vi "Recieve Response with Result.vi"(4 "Finished":bool=TRUE, 6 "Result":refnum<class "Mag Lab Result.lvclass">, 8 "error in (no error)":errorcluster, 9 "Requestor":string, 10 "Requestee":string, 11 "Sequence Stepper in":refnum<class "Sequence Stepper.lvclass">) -> (0 "error out":errorcluster, 3 "Sequence Stepper out":refnum<class "Sequence Stepper.lvclass">)   [LabVIEW 2015, in "Sequence Stepper.lvclass"]
uses:
  Sequence Stepper.lvclass
  Mag Lab Result/Mag Lab Result.lvclass
  Mag Lab Root/Mag Lab Root.lvclass/Mag Lab Root.ctl
  <vilib>/ActorFramework/Actor/Actor.lvclass/Actor.ctl
  Sequence Stepper.lvclass/Sequence Stepper.ctl
  Stepper stage.ctl
  Mag Lab Root Messages/Set Output Msg/Recieve Set Output Msg.lvclass/Recieve Set Output Msg.ctl
  <vilib>/ActorFramework/Message Enqueuer/Message Enqueuer.lvclass/Message Enqueuer.ctl
  <vilib>/ActorFramework/Message Enqueuer/Enqueue.vi
  <vilib>/ActorFramework/Message Priority Queue/Priority Enqueue.vi
  Mag Lab Root Messages/Set Output Msg/Recieve Set Output Msg.lvclass
  Hardware/Source/Settle output/Settle Output.lvclass
  Stepping Function/Stepping Function.lvclass
  Mag Lab Root/Mag Lab Root.lvclass
  <vilib>/ActorFramework/Actor/Actor.lvclass
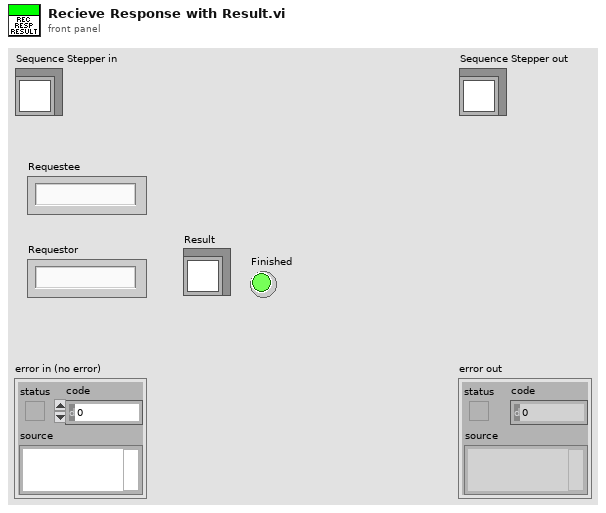
[diagram p1: front panel]
types:
  T1 = typedef "Stepper stage.ctl" = enum16{"New step", "Waiting to settle"}
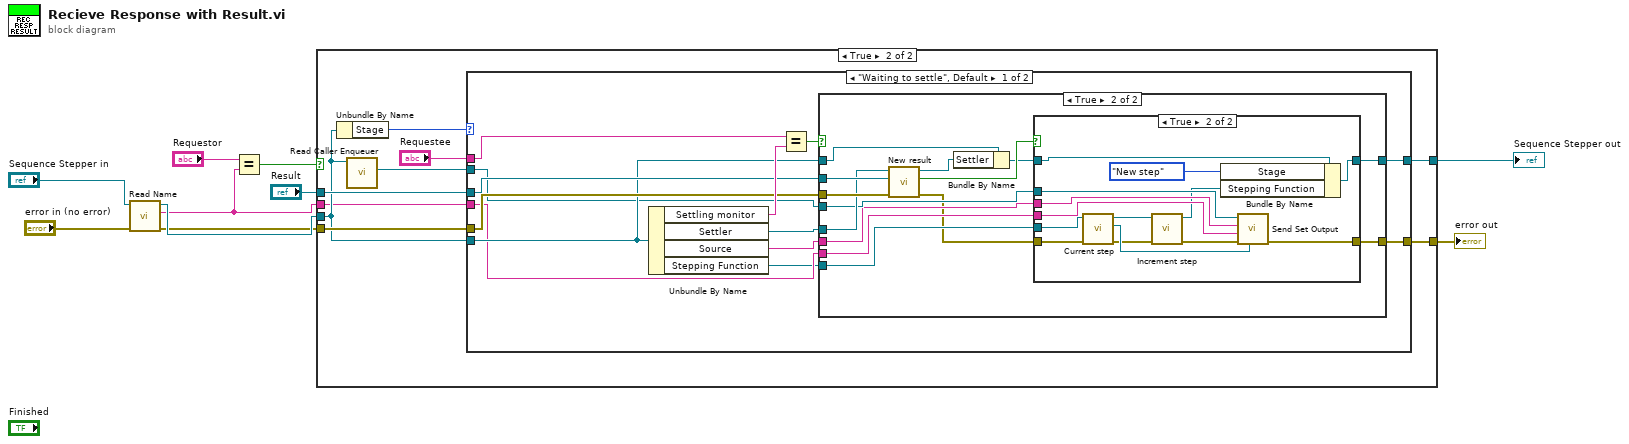
[diagram p0: block diagram]
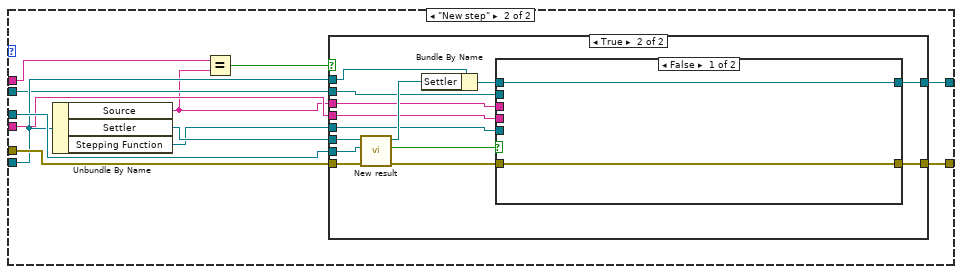
[diagram p5: hidden frame]
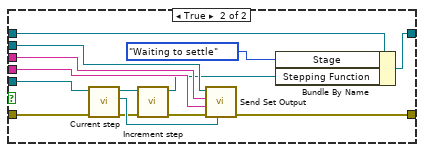
[diagram p7: hidden frame]
diagram:
  n1 = call "Read Name.vi"("error in (no error)"="error in (no error)", "Mag Lab Root in"="Sequence Stepper in") -> ("error out"=w5:errorcluster, "Name"=w3:string, "Mag Lab Root out"=w7:refnum<class "Sequence Stepper.lvclass">)  [unwired: 7 in]
  n2 = Equal?(x="Requestor", y=w3) -> (x = y?=w8:bool)
  n3 = case shown="True" w8 {
    tunnel: w7 -> [w12 w17]
    tunnel: "Result" -> [_ w19]
    tunnel: w5 -> [w11 w18]
    tunnel: w3 -> [_ w15]
    tunnel: [w12 w14] -> w2
    tunnel: [w11 w13] -> w1
    frame False {
    }
    frame True {
      n4 = Unbundle By Name(w17) -> ("Stage"=w21:T1)
      n5 = call <vilib>:"Read Caller Enqueuer.vi"("Actor"=w17) -> ("Caller Enqueuer"=w16:refnum<class "Message Enqueuer.lvclass">)  [unwired: 10 in]
      n6 = case shown="\"Waiting to settle\", Default" w21 {
        tunnel: "Requestee" -> [w34 w78]
        tunnel: w17 -> [w29 w74]
        tunnel: w19 -> [w32 w77]
        tunnel: w18 -> [w31 w76]
        tunnel: w16 -> [w27 w72]
        tunnel: w15 -> [w26 w71]
        tunnel: [w23 w69] -> w14
        tunnel: [w22 w68] -> w13
        frame "Waiting to settle", Default {
          n7 = Unbundle By Name(w29) -> ("Settling monitor"=w33:string, "Settler"=w28:refnum<class "Settle Output.lvclass">, "Source"=w25:string, "Stepping Function"=w24:refnum<class "Stepping Function.lvclass">)
          n8 = Equal?(x=w34, y=w33) -> (x = y?=w30:bool)
          n9 = case shown="True" w30 {
            tunnel: w32 -> [_ w50]
            tunnel: w31 -> [w35 w49]
            tunnel: w29 -> [w36 w48]
            tunnel: w28 -> [_ w46]
            tunnel: w27 -> [_ w43]
            tunnel: w26 -> [_ w42]
            tunnel: w25 -> [_ w41]
            tunnel: w24 -> [_ w40]
            tunnel: [w36 w38] -> w23
            tunnel: [w35 w37] -> w22
            frame False {
            }
            frame True {
              n10 = call-dynamic "New result.vi"("error in (no error)"=w49, "Result"=w50, "Settle Output in"=w46) -> ("error out"=w39:errorcluster, "Is output settled?"=w45:bool, "Settle Output out"=w47:refnum<class "Settle Output.lvclass">)  [unwired: 6 in]
              n11 = Bundle By Name(cluster=w48, "Settler"=w47) -> (w44:refnum<class "Sequence Stepper.lvclass">)
              n12 = case shown="True" w45 {
                tunnel: w44 -> [w52 w66]
                tunnel: w43 -> [_ w64]
                tunnel: w42 -> [_ w62]
                tunnel: w41 -> [_ w63]
                tunnel: w40 -> [_ w61]
                tunnel: w39 -> [w51 w55]
                tunnel: [w52 w54] -> w38
                tunnel: [w51 w53] -> w37
                frame False {
                }
                frame True {
                  n13 = call-dynamic "Current step.vi"("error in (no error)"=w55, "Stepping Function in"=w61) -> ("error out"=w57:errorcluster, "Step value"=w59:refnum<class "Mag Lab Result.lvclass">, "Stepping Function out"=w60:refnum<class "Stepping Function.lvclass">)  [unwired: 7 in]
                  n14 = call-dynamic "Increment step.vi"("error in (no error)"=w57, "Stepping Function in"=w60) -> ("error out"=w56:errorcluster, "Stepping Function out"=w58:refnum<class "Stepping Function.lvclass">)  [unwired: 8 in]
                  n15 = Bundle By Name(cluster=w66, "Stage"=Stepper_stage."New step", "Stepping Function"=w58) -> (w54:refnum<class "Sequence Stepper.lvclass">)
                  n16 = call "Send Set Output.vi"("Output value"=w59, "error in (no error)"=w56, "Requestor"=w62, "Requestee"=w63, "Message Enqueuer"=w64) -> ("error out"=w53:errorcluster)  [unwired: 5 in, 1 out]
                }
              }
            }
          }
        }
        frame "New step" {
          n17 = Unbundle By Name(w74) -> ("Source"=w67:string, "Settler"=w73:refnum<class "Settle Output.lvclass">, "Stepping Function"=w70:refnum<class "Stepping Function.lvclass">)
          n18 = Equal?(x=w78, y=w67) -> (x = y?=w75:bool)
          n19 = case shown="True" w75 {
            tunnel: w77 -> [_ w94]
            tunnel: w76 -> [w79 w93]
            tunnel: w74 -> [w80 w92]
            tunnel: w73 -> [_ w90]
            tunnel: w72 -> [_ w87]
            tunnel: w71 -> [_ w86]
            tunnel: w67 -> [_ w85]
            tunnel: w70 -> [_ w84]
            tunnel: [w80 w82] -> w69
            tunnel: [w79 w81] -> w68
            frame False {
            }
            frame True {
              n20 = call-dynamic "New result.vi"("error in (no error)"=w93, "Result"=w94, "Settle Output in"=w90) -> ("error out"=w83:errorcluster, "Is output settled?"=w89:bool, "Settle Output out"=w91:refnum<class "Settle Output.lvclass">)  [unwired: 6 in]
              n21 = Bundle By Name(cluster=w92, "Settler"=w91) -> (w88:refnum<class "Sequence Stepper.lvclass">)
              n22 = case shown="False" w89 {
                tunnel: w88 -> [w96 w110]
                tunnel: w87 -> [_ w108]
                tunnel: w86 -> [_ w106]
                tunnel: w85 -> [_ w107]
                tunnel: w84 -> [_ w105]
                tunnel: w83 -> [w95 w99]
                tunnel: [w96 w98] -> w82
                tunnel: [w95 w97] -> w81
                frame False {
                }
                frame True {
                  n23 = call-dynamic "Current step.vi"("error in (no error)"=w99, "Stepping Function in"=w105) -> ("error out"=w101:errorcluster, "Step value"=w103:refnum<class "Mag Lab Result.lvclass">, "Stepping Function out"=w104:refnum<class "Stepping Function.lvclass">)  [unwired: 7 in]
                  n24 = call-dynamic "Increment step.vi"("error in (no error)"=w101, "Stepping Function in"=w104) -> ("error out"=w100:errorcluster, "Stepping Function out"=w102:refnum<class "Stepping Function.lvclass">)  [unwired: 8 in]
                  n25 = call "Send Set Output.vi"("Output value"=w103, "error in (no error)"=w100, "Requestor"=w106, "Requestee"=w107, "Message Enqueuer"=w108) -> ("error out"=w97:errorcluster)  [unwired: 5 in, 1 out]
                  n26 = Bundle By Name(cluster=w110, "Stage"=Stepper_stage."Waiting to settle", "Stepping Function"=w102) -> (w98:refnum<class "Sequence Stepper.lvclass">)
                }
              }
            }
          }
        }
      }
    }
  }
  "error out" <- w1
  "Sequence Stepper out" <- w2
